vi "SetRelativePositionUm.vi"(8 "error in (no error)":errorcluster, 9 "RelativeMoveum":dbl min=0.0 max=200.0, 10 "Stage Label":string, 11 "DemoStage in":refnum<class "DemoStage.lvclass">) -> (0 "error out":errorcluster, 3 "DemoStage out":refnum<class "DemoStage.lvclass">)   [LabVIEW 2020, in "DemoStage.lvlib" / "DemoStage.lvclass"]
uses:
  DemoStage.lvclass
  DemoStage.lvclass/DemoStage.ctl
  Hardware Abstraction Layer/Component/Stage/Stage/Stage.lvclass
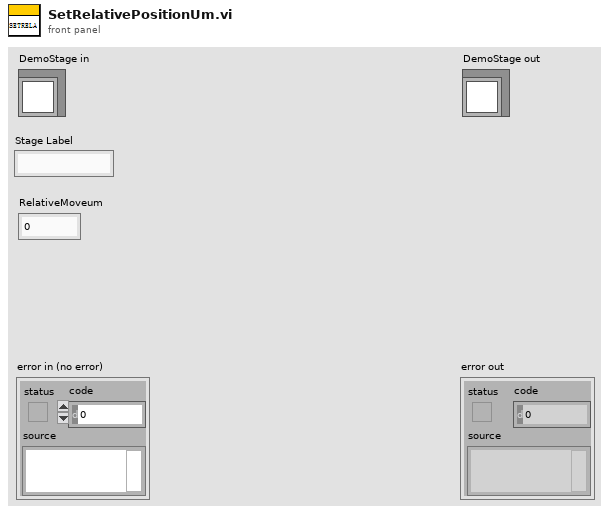
[diagram p1: front panel]
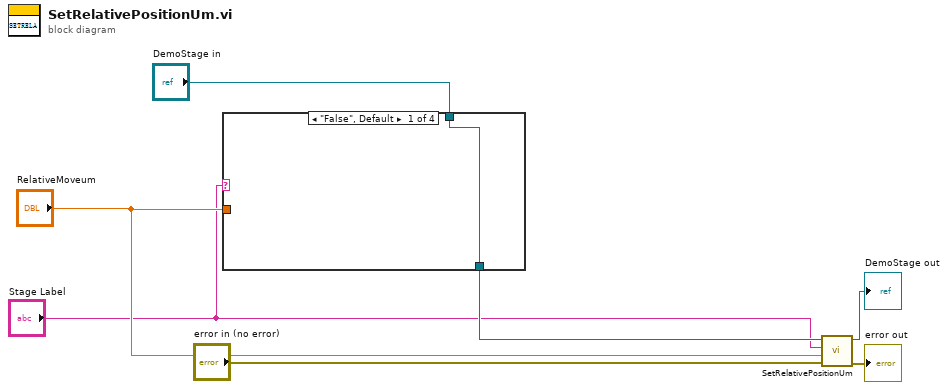
[diagram p0: block diagram]
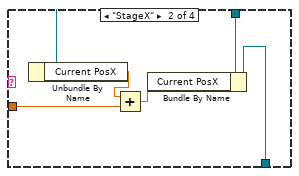
[diagram p2: hidden frame]
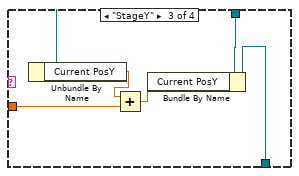
[diagram p3: hidden frame]
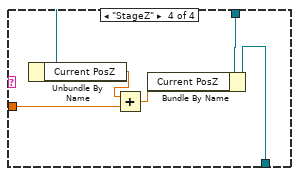
[diagram p4: hidden frame]
diagram:
  n1 = case shown="\"False\", Default" "Stage Label" {
    tunnel: [w8 w13 w18 w23] -> w4
    tunnel: "DemoStage in" -> [w8 w12 w17 w22]
    tunnel: "RelativeMoveum" -> [_ w9 w14 w19]
    frame "False", Default {
    }
    frame "StageX" {
      n2 = Unbundle By Name(w12) -> ("Current PosX"=w11:dbl)
      n3 = Add(x=w11, y=w9) -> (x+y=w10:dbl)
      n4 = Bundle By Name(cluster=w12, "Current PosX"=w10) -> (w13:refnum<class "DemoStage.lvclass">)
    }
    frame "StageY" {
      n5 = Unbundle By Name(w17) -> ("Current PosY"=w16:dbl)
      n6 = Add(x=w16, y=w14) -> (x+y=w15:dbl)
      n7 = Bundle By Name(cluster=w17, "Current PosY"=w15) -> (w18:refnum<class "DemoStage.lvclass">)
    }
    frame "StageZ" {
      n8 = Unbundle By Name(w22) -> ("Current PosZ"=w21:dbl)
      n9 = Add(x=w21, y=w19) -> (x+y=w20:dbl)
      n10 = Bundle By Name(cluster=w22, "Current PosZ"=w20) -> (w23:refnum<class "DemoStage.lvclass">)
    }
  }
  n11 = call-parent "SetRelativePositionUm.vi"("error in (no error)"="error in (no error)", "RelativeMoveum"="RelativeMoveum", "Stage Label"="Stage Label", "Stage in"=w4) -> ("error out"=→"error out":errorcluster, "Stage out"=→"DemoStage out":refnum<class "DemoStage.lvclass">)  [unwired: 6 in]
